vi "Execute Command.vi"(0 "Session Handle in":T1, 5 "resources":string, 7 "command":refnum<k21>, 11 "error in (no error)":errorcluster) -> (4 "Session Handle out":T1, 15 "error out":errorcluster)   [LabVIEW 2015, in "SLSC Switch.lvlib" / "SLSC Session.lvclass"]
uses:
  SLSC Session.lvclass
  Typedefs/Session Handle.ctl
  SLSC Session.lvclass/SLSC Session.ctl
  <vilib>/SLSC/SLSC.lvlib
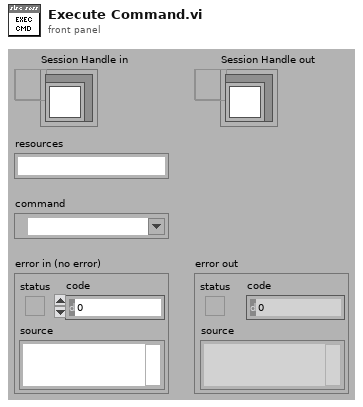
[diagram p1: front panel]
types:
  T1 = typedef "SLSC Switch.lvlib/SLSC Session.lvclass/Session Handle.ctl" = refnum<data-value>
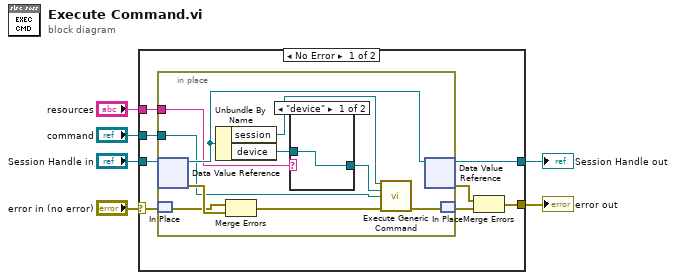
[diagram p0: block diagram]
diagram:
  n1 = case shown="No Error" "error in (no error)" {
    selector: "error in (no error)" -> [w9 w27]
    tunnel: "Session Handle in" -> [w14 w28]
    tunnel: [w13 w28] -> w5
    tunnel: [w10 w27] -> w4
    tunnel: "command" -> [w8 _]
    tunnel: "resources" -> [w7 _]
    frame No Error {
      n2 = in-place {
        in-place-border: w8 -> [w20]
        in-place-border: w7 -> [w17]
        n3 = in-place-dvr #1(w14) -> (w22:refnum<class "SLSC Session.lvclass">, w24:errorcluster)
        n4 = in-place-match #2(w9) -> (w23:errorcluster)
        n5 = Unbundle By Name(w22) -> ("session"=w21:refnum<k21>, "device"=w15:refnum<k21>)
        n6 = Merge Errors(w23, w24) -> (w19:errorcluster)
        n7 = case shown="\"device\"" w17 {
          selector: w17 -> [_ w26]
          tunnel: [w25 w26] -> w16
          tunnel: w15 -> [w25 _]
          frame "device" {
          }
          frame Default {
          }
        }
        n8 = call <vilib>:"Execute Generic Command.vi"("session in"=w21, "resources"=w16, "command"=w20, "error in (no error)"=w19) -> ("error out"=w18:errorcluster)  [unwired: 10 in, 1 out]
        n9 = in-place-dvr #1(w22) -> (w13:T1, w11:errorcluster)
        n10 = in-place-match #2(w18) -> (w12:errorcluster)
      }
      n11 = Merge Errors(w11, w12) -> (w10:errorcluster)
    }
    frame Error {
    }
  }
  "Session Handle out" <- w5
  "error out" <- w4
